vi "Teleop V2.vi"   [LabVIEW 2018]
uses:
  <vilib>/Rock Robotics/WPI/Solenoid/WPI_SolenoidValue.ctl
  Various Globals.vi
  Refnums.vi
  <vilib>/Rock Robotics/Network Tables/NT Write Number.vi
  <vilib>/Rock Robotics/WPI/Solenoid/WPI_SolenoidSetEnum.vi
  Positions.vi
  <vilib>/Rock Robotics/WPI/RobotDrive/WPI_RobotDriveArcadeDrive_Standard(NoSaturation).vi
types:
  T1 = typedef "WPI_SolenoidValue.ctl" = enum16{"Off", "On", "Forward", "Reverse"}
  T2 = typedef "WPI_JoystickDevRef.ctl" = cluster{"Device":T3}
  T3 = typedef "WPI_JoystickDeviceEnum.ctl" = enum16{"USB 0", "USB 1", "USB 2", "USB 3", "USB 4", "USB 5"}
  T4 = typedef "WPI_SolenoidDevRef.ctl" = cluster{"DevStatus":errorcluster, "Pneumatics Control Module":u8, "Forward Solenoid Channel":T5, "Reverse Solenoid Channel":T5}
  T5 = typedef "WPI_SolenoidChannel.ctl" = enum8{"Solenoid 0", "Solenoid 1", "Solenoid 2", "Solenoid 3", "Solenoid 4", "Solenoid 5", "Solenoid 6", "Solenoid 7", "Invalid"}
  T6 = typedef "WPI_CompressorDevRef.ctl" = cluster{"DevStatus":errorcluster, "Pneumatics Control Module":u8}
  T7 = cluster{"DriveShifter":T4, "Ouput":T4, "Compressor":T6, "Climb Piston":T4}
  T8 = typedef "WPI_DigitalInputDevRef.ctl" = cluster{"DevStatus":errorcluster, "DIO Channel":T9}
  T9 = typedef "FPGA_DIOChannel.ctl" = enum8{"DIO 0", "DIO 1", "DIO 2", "DIO 3", "DIO 4", "DIO 5", "DIO 6", "DIO 7", "DIO 8", "DIO 9", "DIO MXP 0", "DIO MXP 1", "DIO MXP 2", "DIO MXP 3", "DIO MXP 4", "DIO MXP 5", "DIO MXP 6", "DIO MXP 7", "DIO MXP 8", "DIO MXP 9", "DIO MXP 10", "DIO MXP 11", "DIO MXP 12", "DIO MXP 13", "DIO MXP 14", "DIO MXP 15", "SPI Port CS1", "SPI Port CS2", "SPI Port CS3", "SPI Port MISO", "SPI Port MOSI", "Invalid"}
  T10 = typedef "WPI_RobotDriveDevRef.ctl" = cluster{"DevStatus":errorcluster, "Motors[]":T11[], "Square Inputs":bool, "Max Output":dbl}
  T11 = typedef "WPI_MotorControlDeviceRef.ctl" = cluster{"DeviceStatus":errorcluster, "Type":T12, "PWM":cluster{"PWM Channel":T13, "DeadBand":T14}, "CAN":cluster{"Device Number":u8, "SetOutput VI Ref":variant, "GetOutput VI Ref":variant, "Enable VI Ref":variant, "Disable VI Ref":variant, "Data":variant}, "Invert":bool, "DIO PWM":cluster{"PWM \"Enable\" Channel":T13, "DIOChannel":T9, "PWM Rate":dbl}}
  T12 = typedef "WPI_MotorControlType.ctl" = enum16{"PWM", "CAN", "DIO PWM"}
  T13 = typedef "FPGA_DIOPWMChannel.ctl" = enum8{"PWM 0", "PWM 1", "PWM 2", "PWM 3", "PWM 4", "PWM 5", "PWM 6", "PWM 7", "PWM 8", "PWM 9", "PWM MXP 0", "PWM MXP 1", "PWM MXP 2", "PWM MXP 3", "PWM MXP 4", "PWM MXP 5", "PWM MXP 6", "PWM MXP 7", "PWM MXP 8", "PWM MXP 9", "Invalid"}
  T14 = typedef "WPI_PWMDeadband.ctl" = cluster{"Name":string, "maxPositivePwm":i32, "minPositivePwm":i32, "centerPwm":i32, "maxNegativePwm":i32, "minNegativePwm":i32, "angularRange":u16}
  T15 = cluster{"DriveTrain":T10, "LeftDrive":T11, "RightDrive":T11, "Elevator":T11, "Pivot":T11, "Intake":T11, "Right Climber":T11, "Left Climber":T11, "Shooter":T11}
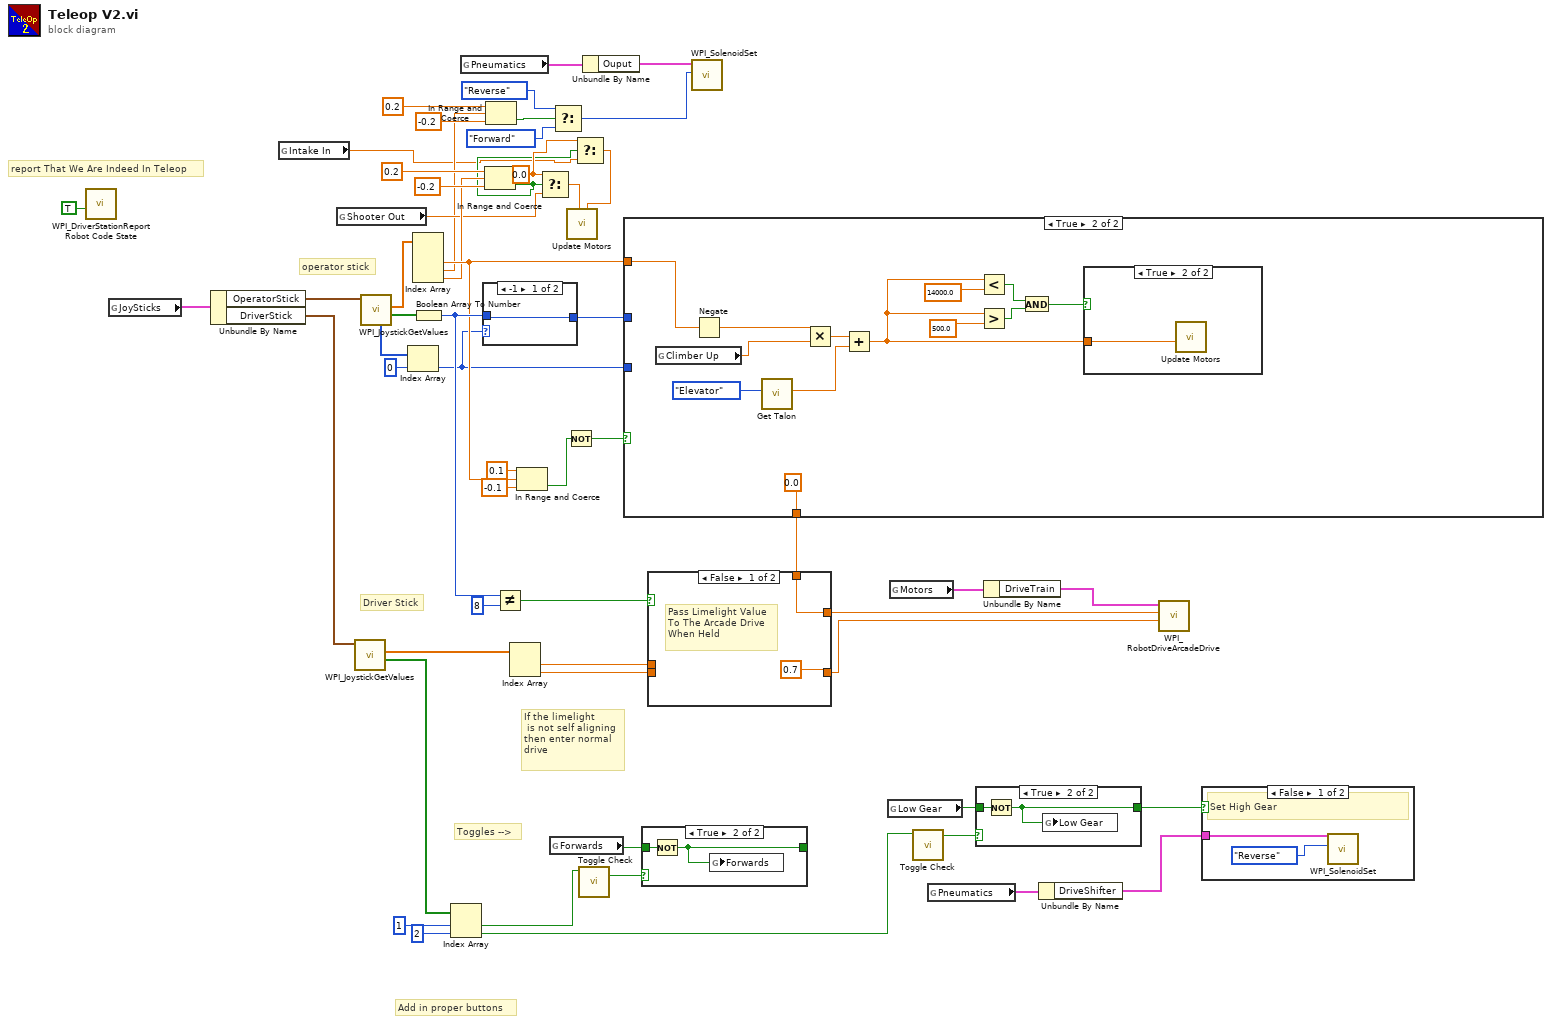
[diagram p0: block diagram]
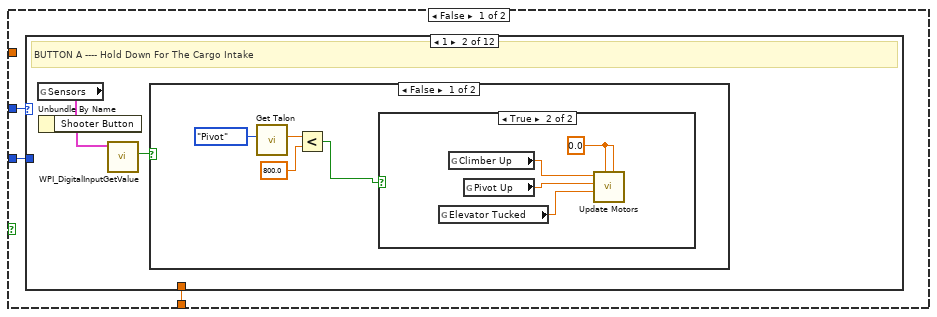
[diagram p2: hidden frame]
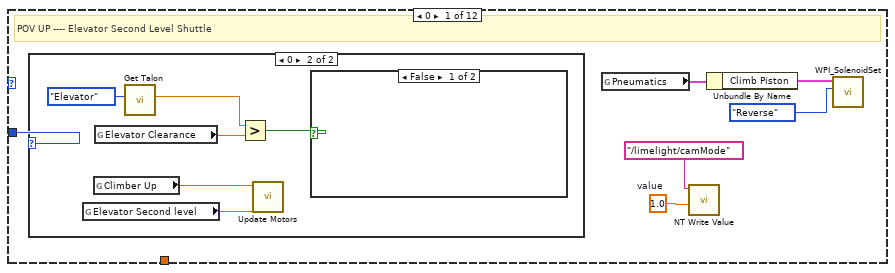
[diagram p3: hidden frame]
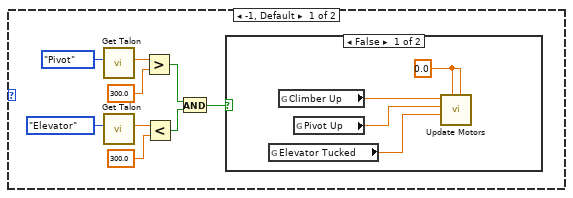
[diagram p4: hidden frame]
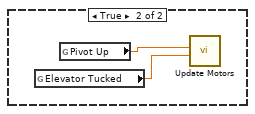
[diagram p5: hidden frame]
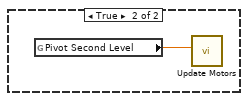
[diagram p6: hidden frame]
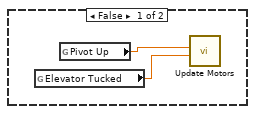
[diagram p7: hidden frame]
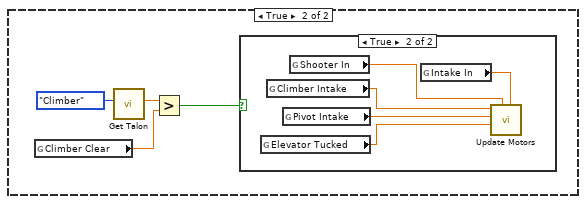
[diagram p8: hidden frame]
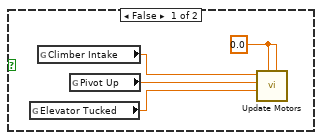
[diagram p9: hidden frame]
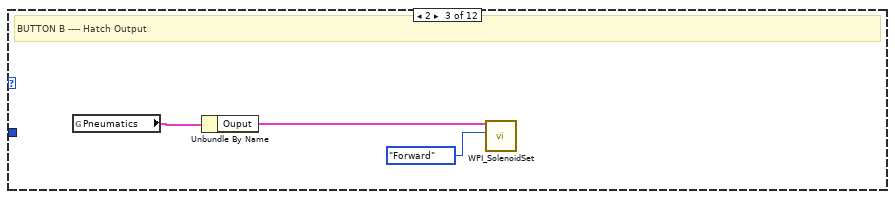
[diagram p10: hidden frame]
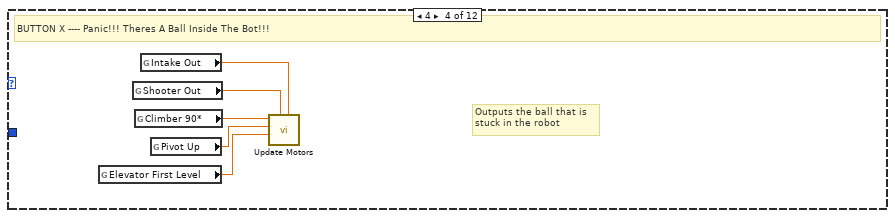
[diagram p11: hidden frame]
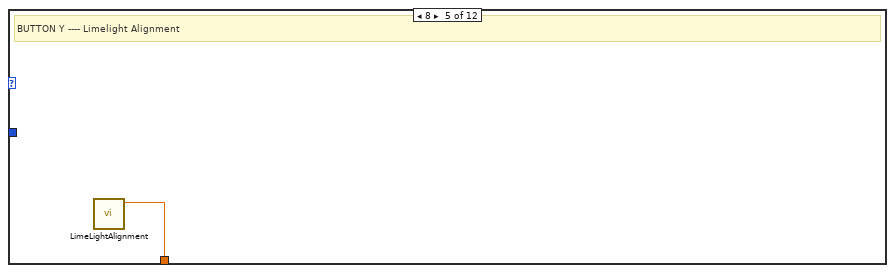
[diagram p12: hidden frame]
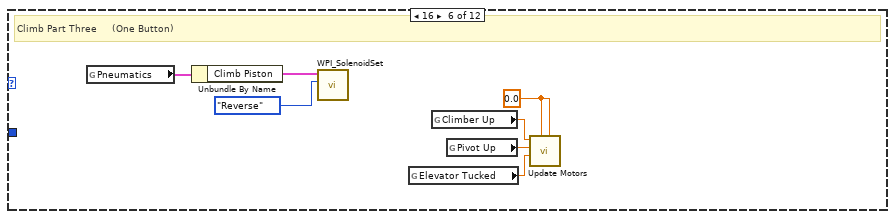
[diagram p13: hidden frame]
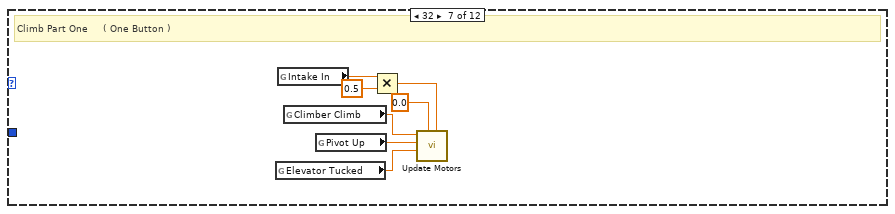
[diagram p14: hidden frame]
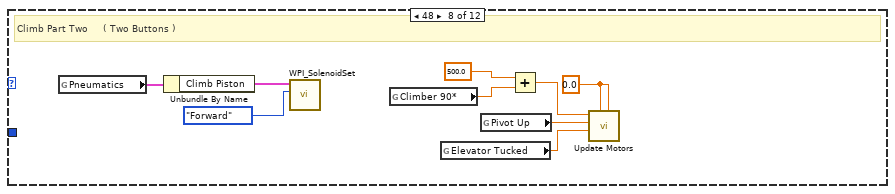
[diagram p15: hidden frame]
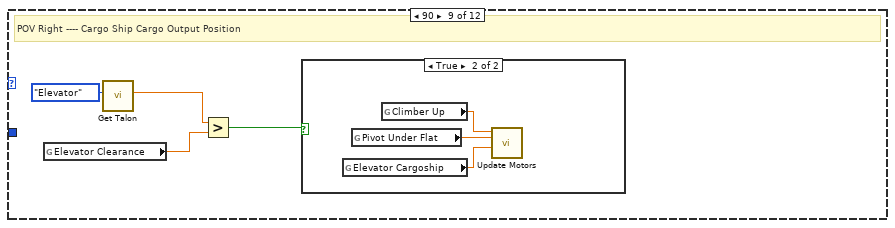
[diagram p16: hidden frame]
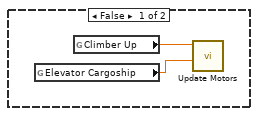
[diagram p17: hidden frame]
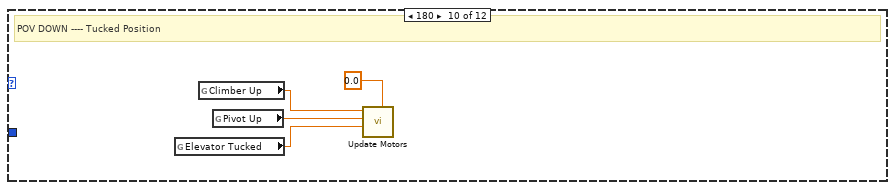
[diagram p18: hidden frame]
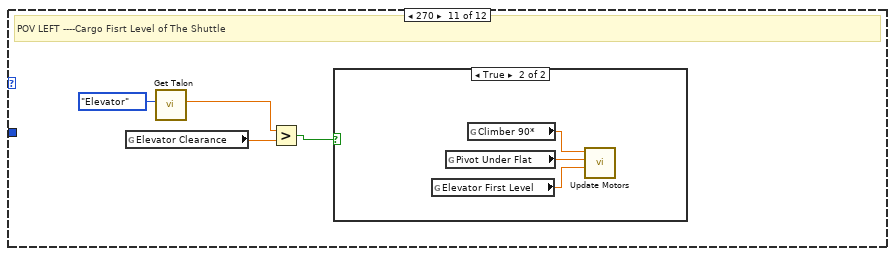
[diagram p19: hidden frame]
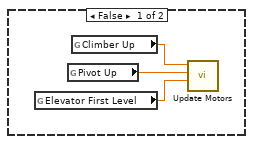
[diagram p20: hidden frame]
diagram:
  w6 = 0.0 ("t")
  # "report That We Are Indeed In Teleop"
  # "operator stick"
  # "Driver Stick"
  # "Add in proper buttons"
  # "Toggles -->"
  # "If the limelight\n is not self aligning\nthen enter normal \ndrive"
  n1 = call <vilib>:"WPI_DriverStationReport Robot Code State.vi"("TeleOp"=TRUE ("Autonomous")) -> ()  [unwired: 10 in, 1 out]
  n2 = global read "Refnums.vi" "JoySticks"() -> (w41:cluster{"DriverStick":T2, "OperatorStick":T2})
  n3 = Unbundle By Name(w41) -> ("OperatorStick"=w40:T2, "DriverStick"=w39:T2)
  n4 = global read "Positions.vi" "Intake In"() -> (w3:dbl)
  n5 = global read "Positions.vi" "Shooter Out"() -> (w17:dbl)
  n6 = call <vilib>:"WPI_JoystickGetValues.vi"("JoystickDevRef"=w39) -> ("Buttons"=w54:bool[], "Axes"=w45:dbl[])  [unwired: 6 in, 3 out]
  n7 = call <vilib>:"WPI_JoystickGetValues.vi"("JoystickDevRef"=w40) -> ("Buttons"=w42:bool[], "Axes"=w35:dbl[], "POVs"=w31:i16[])  [unwired: 6 in, 2 out]
  n8 = Index Array(array=w31, index=0) -> (element=w22:i16)
  n9 = Index Array(array=w35) -> (element #2=w26:dbl, element #3=w14:dbl, element #4=w19:dbl)  [unwired: 4 in, 1 out]
  n10 = Boolean Array To Number(Boolean array=w42) -> (number=w29:u32)
  n11 = Index Array(array=w54, index #1=1 ("index"), index #2=2 ("index")) -> (element #1=w53:bool, element #2=w50:bool)
  n12 = global read "Refnums.vi" "Pneumatics"() -> (w12:T7)
  n13 = case shown="-1" w22 {
    selector: w22 -> [_ w59]
    tunnel: w29 -> [w57 w60]
    tunnel: [w57 w58] -> w27
    frame -1 {
    }
    frame Default {
      n14 = Add(x=w60, y=w59) -> (x+y=w58:u32)
    }
  }
  n15 = In Range and Coerce(upper limit=0.2, x=w19, lower limit=-0.2) -> (In Range?=w5:bool)  [unwired: 1 out]
  n16 = In Range and Coerce(upper limit=0.2, x=w14, lower limit=-0.2) -> (In Range?=w13:bool)  [unwired: 1 out]
  n17 = Not Equal?(x=w29, y=u32 8) -> (x != y?=w2:bool)
  n18 = Index Array(array=w45) -> (element #1=w44:dbl, element #2=w43:dbl)  [unwired: 2 in]
  n19 = In Range and Coerce(upper limit=0.1, x=w26, lower limit=-0.1) -> (In Range?=w18:bool)  [unwired: 1 out]
  n20 = Select(t=w6, s=w5, f=w17) -> (s? t:f=w7:dbl)
  n21 = global read "Various Globals.vi" "Forwards"() -> (w55:bool)
  n22 = Select(t=WPI_SolenoidValue."Reverse" ("Value"), s=w13, f=WPI_SolenoidValue."Forward" ("Value")) -> (s? t:f=w8:T1)
  n23 = Not(x=w18) -> (.not. x?=w23:bool)
  n24 = Select(t=w6, s=w5, f=w3) -> (s? t:f=w4:dbl)
  n25 = call "Update Motors.vi"("Intake"=w4, "Shooter"=w7) -> ()  [unwired: 10 in]
  n26 = call "Toggle Check.vi"("button in"=w53) -> ("toggled?"=w56:bool)  [unwired: 10 in]
  n27 = Unbundle By Name(w12) -> ("Ouput"=w11:T4)
  n28 = case shown="True" w23 {
    tunnel: [w61 0.0] -> w47
    tunnel: w26 -> [_ w179]
    tunnel: w27 -> [w63 _]
    tunnel: w22 -> [w62 _]
    frame False {
      n29 = case shown="1" w63 {
        tunnel: w62 -> [w69 _ _ _ _ _ _ _ _ _ _ _]
        tunnel: [_ _ _ _ w126 _ _ _ _ _ _ _] -> w61
        frame 0 {
          w67 = 1.0  # value
          # "POV UP ---- Elevator Second Level Shuttle"
          n30 = case shown="0" w69 {
            frame -1, Default {
              n31 = call "Get Talon.vi"("Enum"=enum16{"Climber", "Elevator", "Pivot"}."Pivot") -> ("Position"=w76:dbl)  [unwired: 10 in]
              n32 = call "Get Talon.vi"("Enum"=enum16{"Climber", "Elevator", "Pivot"}."Elevator") -> ("Position"=w74:dbl)  [unwired: 10 in]
              n33 = Greater?(x=w76, y=300.0) -> (0:w71:bool)
              n34 = Less?(x=w74, y=300.0) -> (x < y?=w72:bool)
              n35 = And(x=w71, y=w72) -> (x .and. y?=w70:bool)
              n36 = case shown="False" w70 {
                frame False {
                  w79 = 0.0 ("Shooter")
                  n37 = global read "Positions.vi" "Elevator Tucked"() -> (w81:dbl)
                  n38 = global read "Positions.vi" "Climber Up"() -> (w80:dbl)
                  n39 = global read "Positions.vi" "Pivot Up"() -> (w82:dbl)
                  n40 = call "Update Motors.vi"("Intake"=w79, "Shooter"=w79, "Elevator"=w81, "Pivot"=w82, "Climber"=w80) -> ()  [unwired: 7 in]
                }
                frame True {
                  n41 = global read "Positions.vi" "Elevator Tucked"() -> (w83:dbl)
                  n42 = global read "Positions.vi" "Pivot Up"() -> (w84:dbl)
                  n43 = call "Update Motors.vi"("Elevator"=w83, "Pivot"=w84) -> ()  [unwired: 10 in]
                }
              }
            }
            frame 0 {
              n44 = global read "Positions.vi" "Elevator Second level"() -> (w86:dbl)
              n45 = global read "Positions.vi" "Climber Up"() -> (w85:dbl)
              n46 = global read "Positions.vi" "Elevator Clearance"() -> (w88:dbl)
              n47 = call "Get Talon.vi"("Enum"=enum16{"Climber", "Elevator", "Pivot"}."Elevator") -> ("Position"=w87:dbl)  [unwired: 10 in]
              n48 = Greater?(x=w87, y=w88) -> (0:w89:bool)
              n49 = call "Update Motors.vi"("Elevator"=w86, "Climber"=w85) -> ()  [unwired: 10 in]
              n50 = case shown="False" w89 {
                frame False {
                }
                frame True {
                  n51 = global read "Positions.vi" "Pivot Second Level"() -> (w91:dbl)
                  n52 = call "Update Motors.vi"("Pivot"=w91) -> ()  [unwired: 11 in]
                }
              }
            }
          }
          n53 = global read "Refnums.vi" "Pneumatics"() -> (w66:T7)
          n54 = call-poly <vilib>:"NT Write Value.vi"("Numeric"=w67, "Name"="/limelight/camMode") -> ()  [unwired: 9 in, 1 out]
          n55 = Unbundle By Name(w66) -> ("Climb Piston"=w65:T4)
          n56 = call-poly <vilib>:"WPI_SolenoidSet.vi"("Value"=WPI_SolenoidValue."Reverse", "SolenoidDevRef"=w65) -> ()  [unwired: 8 in, 2 out]
        }
        frame 1 {
          # "BUTTON A ---- Hold Down For The Cargo Intake"
          n57 = global read "Refnums.vi" "Sensors"() -> (w94:cluster{"Shooter Button":T8})
          n58 = Unbundle By Name(w94) -> ("Shooter Button"=w93:T8)
          n59 = call <vilib>:"WPI_DigitalInputGetValue.vi"("DigitalInputDevRef"=w93) -> ("Value"=w92:bool)  [unwired: 8 in, 2 out]
          n60 = case shown="False" w92 {
            frame False {
              n61 = call "Get Talon.vi"("Enum"=enum16{"Climber", "Elevator", "Pivot"}."Pivot") -> ("Position"=w97:dbl)  [unwired: 10 in]
              n62 = Less?(x=w97, y=800.0) -> (x < y?=w95:bool)
              n63 = case shown="True" w95 {
                frame False {
                  n64 = global read "Positions.vi" "Elevator Tucked"() -> (w99:dbl)
                  n65 = global read "Positions.vi" "Pivot Up"() -> (w100:dbl)
                  n66 = call "Update Motors.vi"("Elevator"=w99, "Pivot"=w100) -> ()  [unwired: 10 in]
                }
                frame True {
                  w101 = 0.0 ("Shooter")
                  n67 = global read "Positions.vi" "Elevator Tucked"() -> (w103:dbl)
                  n68 = global read "Positions.vi" "Climber Up"() -> (w102:dbl)
                  n69 = global read "Positions.vi" "Pivot Up"() -> (w104:dbl)
                  n70 = call "Update Motors.vi"("Intake"=w101, "Shooter"=w101, "Elevator"=w103, "Pivot"=w104, "Climber"=w102) -> ()  [unwired: 7 in]
                }
              }
            }
            frame True {
              n71 = global read "Positions.vi" "Climber Clear"() -> (w105:dbl)
              n72 = call "Get Talon.vi"("Enum"=enum16{"Climber", "Elevator", "Pivot"}."Climber") -> ("Position"=w107:dbl)  [unwired: 10 in]
              n73 = Greater?(x=w107, y=w105) -> (0:w106:bool)
              n74 = case shown="True" w106 {
                frame False {
                  w109 = 0.0 ("Shooter")
                  n75 = global read "Positions.vi" "Elevator Tucked"() -> (w111:dbl)
                  n76 = global read "Positions.vi" "Climber Intake"() -> (w110:dbl)
                  n77 = global read "Positions.vi" "Pivot Up"() -> (w112:dbl)
                  n78 = call "Update Motors.vi"("Intake"=w109, "Shooter"=w109, "Elevator"=w111, "Pivot"=w112, "Climber"=w110) -> ()  [unwired: 7 in]
                }
                frame True {
                  n79 = global read "Positions.vi" "Elevator Tucked"() -> (w116:dbl)
                  n80 = global read "Positions.vi" "Climber Intake"() -> (w115:dbl)
                  n81 = global read "Positions.vi" "Pivot Intake"() -> (w117:dbl)
                  n82 = global read "Positions.vi" "Shooter In"() -> (w114:dbl)
                  n83 = global read "Positions.vi" "Intake In"() -> (w113:dbl)
                  n84 = call "Update Motors.vi"("Intake"=w113, "Shooter"=w114, "Elevator"=w116, "Pivot"=w117, "Climber"=w115) -> ()  [unwired: 7 in]
                }
              }
            }
          }
        }
        frame 2 {
          # "BUTTON B ---- Hatch Output"
          n85 = global read "Refnums.vi" "Pneumatics"() -> (w120:T7)
          n86 = Unbundle By Name(w120) -> ("Ouput"=w118:T4)
          n87 = call-poly <vilib>:"WPI_SolenoidSet.vi"("Value"=WPI_SolenoidValue."Forward", "SolenoidDevRef"=w118) -> ()  [unwired: 8 in, 2 out]
        }
        frame 4 {
          # "Outputs the ball that is \nstuck in the robot"
          # "BUTTON X ---- Panic!!! Theres A Ball Inside The Bot!!!"
          n88 = global read "Positions.vi" "Elevator First Level"() -> (w123:dbl)
          n89 = global read "Positions.vi" "Shooter Out"() -> (w122:dbl)
          n90 = global read "Positions.vi" "Climber 90*"() -> (w125:dbl)
          n91 = global read "Positions.vi" "Intake Out"() -> (w121:dbl)
          n92 = global read "Positions.vi" "Pivot Up"() -> (w124:dbl)
          n93 = call "Update Motors.vi"("Intake"=w121, "Shooter"=w122, "Elevator"=w123, "Pivot"=w124, "Climber"=w125) -> ()  [unwired: 7 in]
        }
        frame 8 {
          # "BUTTON Y ---- Limelight Alignment"
          n94 = call "LimeLightAlignment.vi"() -> ("Correction"=w126:dbl)  [unwired: 9 in, 1 out]
        }
        frame 16 {
          w127 = 0.0 ("Shooter")
          # "Climb Part Three     (One Button)"
          n95 = global read "Refnums.vi" "Pneumatics"() -> (w133:T7)
          n96 = Unbundle By Name(w133) -> ("Climb Piston"=w132:T4)
          n97 = call-poly <vilib>:"WPI_SolenoidSet.vi"("Value"=WPI_SolenoidValue."Reverse", "SolenoidDevRef"=w132) -> ()  [unwired: 8 in, 2 out]
          n98 = global read "Positions.vi" "Elevator Tucked"() -> (w128:dbl)
          n99 = global read "Positions.vi" "Climber Up"() -> (w130:dbl)
          n100 = global read "Positions.vi" "Pivot Up"() -> (w129:dbl)
          n101 = call "Update Motors.vi"("Intake"=w127, "Shooter"=w127, "Elevator"=w128, "Pivot"=w129, "Climber"=w130) -> ()  [unwired: 7 in]
        }
        frame 32 {
          # "Climb Part One     ( One Button )"
          n102 = global read "Positions.vi" "Elevator Tucked"() -> (w138:dbl)
          n103 = global read "Positions.vi" "Intake In"() -> (w137:dbl)
          n104 = global read "Positions.vi" "Climber Climb"() -> (w140:dbl)
          n105 = global read "Positions.vi" "Pivot Up"() -> (w139:dbl)
          n106 = Multiply(x=w137, y=0.5) -> (x*y=w135:dbl)
          n107 = call "Update Motors.vi"("Intake"=w135, "Shooter"=0.0, "Elevator"=w138, "Pivot"=w139, "Climber"=w140) -> ()  [unwired: 7 in]
        }
        frame 48 {
          w141 = 0.0 ("Shooter")
          # "Climb Part Two     ( Two Buttons )"
          n108 = global read "Refnums.vi" "Pneumatics"() -> (w149:T7)
          n109 = Unbundle By Name(w149) -> ("Climb Piston"=w148:T4)
          n110 = call-poly <vilib>:"WPI_SolenoidSet.vi"("Value"=WPI_SolenoidValue."Forward", "SolenoidDevRef"=w148) -> ()  [unwired: 8 in, 2 out]
          n111 = global read "Positions.vi" "Climber 90*"() -> (w143:dbl)
          n112 = global read "Positions.vi" "Elevator Tucked"() -> (w145:dbl)
          n113 = global read "Positions.vi" "Pivot Up"() -> (w146:dbl)
          n114 = Add(x=500.0, y=w143) -> (x+y=w144:dbl)
          n115 = call "Update Motors.vi"("Intake"=w141, "Shooter"=w141, "Elevator"=w145, "Pivot"=w146, "Climber"=w144) -> ()  [unwired: 7 in]
        }
        frame 90 {
          # "POV Right ---- Cargo Ship Cargo Output Position"
          n116 = global read "Positions.vi" "Elevator Clearance"() -> (w150:dbl)
          n117 = call "Get Talon.vi"("Enum"=enum16{"Climber", "Elevator", "Pivot"}."Elevator") -> ("Position"=w152:dbl)  [unwired: 10 in]
          n118 = Greater?(x=w152, y=w150) -> (0:w151:bool)
          n119 = case shown="True" w151 {
            frame False {
              n120 = global read "Positions.vi" "Elevator Cargoship"() -> (w155:dbl)
              n121 = global read "Positions.vi" "Climber Up"() -> (w154:dbl)
              n122 = call "Update Motors.vi"("Elevator"=w155, "Climber"=w154) -> ()  [unwired: 10 in]
            }
            frame True {
              n123 = global read "Positions.vi" "Elevator Cargoship"() -> (w158:dbl)
              n124 = global read "Positions.vi" "Pivot Under Flat"() -> (w157:dbl)
              n125 = global read "Positions.vi" "Climber Up"() -> (w156:dbl)
              n126 = call "Update Motors.vi"("Elevator"=w158, "Pivot"=w157, "Climber"=w156) -> ()  [unwired: 9 in]
            }
          }
        }
        frame 180 {
          # "POV DOWN ---- Tucked Position"
          n127 = global read "Positions.vi" "Elevator Tucked"() -> (w160:dbl)
          n128 = global read "Positions.vi" "Climber Up"() -> (w162:dbl)
          n129 = global read "Positions.vi" "Pivot Up"() -> (w161:dbl)
          n130 = call "Update Motors.vi"("Intake"=0.0, "Elevator"=w160, "Pivot"=w161, "Climber"=w162) -> ()  [unwired: 8 in]
        }
        frame 270 {
          # "POV LEFT ----Cargo Fisrt Level of The Shuttle"
          n131 = global read "Positions.vi" "Elevator Clearance"() -> (w165:dbl)
          n132 = call "Get Talon.vi"("Enum"=enum16{"Climber", "Elevator", "Pivot"}."Elevator") -> ("Position"=w164:dbl)  [unwired: 10 in]
          n133 = Greater?(x=w164, y=w165) -> (0:w163:bool)
          n134 = case shown="True" w163 {
            frame False {
              n135 = global read "Positions.vi" "Elevator First Level"() -> (w167:dbl)
              n136 = global read "Positions.vi" "Pivot Up"() -> (w169:dbl)
              n137 = global read "Positions.vi" "Climber Up"() -> (w168:dbl)
              n138 = call "Update Motors.vi"("Elevator"=w167, "Pivot"=w169, "Climber"=w168) -> ()  [unwired: 9 in]
            }
            frame True {
              n139 = global read "Positions.vi" "Elevator First Level"() -> (w170:dbl)
              n140 = global read "Positions.vi" "Pivot Under Flat"() -> (w172:dbl)
              n141 = global read "Positions.vi" "Climber 90*"() -> (w171:dbl)
              n142 = call "Update Motors.vi"("Elevator"=w170, "Pivot"=w172, "Climber"=w171) -> ()  [unwired: 9 in]
            }
          }
        }
        frame Default {
        }
      }
    }
    frame True {
      n143 = global read "Positions.vi" "Climber Up"() -> (w173:dbl)
      n144 = Negate(x=w179) -> (-x=w178:dbl)
      n145 = call "Get Talon.vi"("Enum"=enum16{"Climber", "Elevator", "Pivot"}."Elevator") -> ("Position"=w180:dbl)  [unwired: 10 in]
      n146 = Multiply(x=w178, y=w173) -> (x*y=w181:dbl)
      n147 = Add(x=w181, y=w180) -> (x+y=w182:dbl)
      n148 = Less?(x=w182, y=14000.0) -> (x < y?=w174:bool)
      n149 = Greater?(x=w182, y=500.0) -> (0:w176:bool)
      n150 = And(x=w174, y=w176) -> (x .and. y?=w175:bool)
      n151 = case shown="True" w175 {
        tunnel: w182 -> [_ w186]
        frame False {
        }
        frame True {
          n152 = call "Update Motors.vi"("Elevator"=w186) -> ()  [unwired: 11 in]
        }
      }
    }
  }
  n153 = case shown="True" w56 {
    tunnel: [w187 w189] -> _
    tunnel: w55 -> [w187 w188]
    frame False {
    }
    frame True {
      n154 = Not(x=w188) -> (.not. x?=w189:bool)
      n155 = global write "Various Globals.vi" "Forwards"(w189) -> ()
    }
  }
  n156 = case shown="False" w2 {
    tunnel: w47 -> [w191 _]
    tunnel: [w191 w193] -> w46
    tunnel: w44 -> [_ w192]
    tunnel: [0.7 w194] -> w1
    tunnel: w43 -> [_ w194]
    frame False {
      # "Pass Limelight Value\nTo The Arcade Drive\nWhen Held"
    }
    frame True {
      # "Normal Drive"
      n157 = Negate(x=w192) -> (-x=w193:dbl)
    }
  }
  n158 = call-poly <vilib>:"WPI_SolenoidSet.vi"("Value"=w8, "SolenoidDevRef"=w11) -> ()  [unwired: 8 in, 2 out]
  n159 = global read "Various Globals.vi" "Low Gear"() -> (w51:bool)
  n160 = global read "Refnums.vi" "Motors"() -> (w33:T15)
  n161 = call "Toggle Check.vi"("button in"=w50) -> ("toggled?"=w52:bool)  [unwired: 10 in]
  n162 = global read "Refnums.vi" "Pneumatics"() -> (w36:T7)
  n163 = case shown="True" w52 {
    tunnel: [w195 w197] -> w49
    tunnel: w51 -> [w195 w196]
    frame False {
    }
    frame True {
      n164 = Not(x=w196) -> (.not. x?=w197:bool)
      n165 = global write "Various Globals.vi" "Low Gear"(w197) -> ()
    }
  }
  n166 = Unbundle By Name(w33) -> ("DriveTrain"=w32:T10)
  n167 = Unbundle By Name(w36) -> ("DriveShifter"=w34:T4)
  n168 = call-poly <vilib>:"WPI_RobotDriveArcadeDrive.vi"("Y axis value"=w1, "X axis value"=w46, "RobotDriveDevRef"=w32) -> ()  [unwired: 6 in, 3 out]
  n169 = case shown="False" w49 {
    tunnel: w34 -> [w198 w200]
    frame False {
      # "Set High Gear"
      n170 = call-poly <vilib>:"WPI_SolenoidSet.vi"("Value"=WPI_SolenoidValue."Reverse", "SolenoidDevRef"=w198) -> ()  [unwired: 8 in, 2 out]
    }
    frame True {
      # "Set  Low Gear"
      n171 = call-poly <vilib>:"WPI_SolenoidSet.vi"("Value"=WPI_SolenoidValue."Forward", "SolenoidDevRef"=w200) -> ()  [unwired: 8 in, 2 out]
    }
  }
